vi "Gas_Release_Control.vi"(4 "Source Establishment Time (s)":dbl=20.0, 5 "Gas Line Name":T1, 6 "Strength (% by volume)":dbl format="%.3f", 7 "Carrier_2 Q (l/min)":dbl format="%.2f", 8 "Carrier_1 Q (l/min)":dbl format="%#.3f", 9 "Source Status":T3=enum."Using") -> (0 "error out":errorcluster, 1 "Flowrates (kg/min)":dbl[](array[numeric]) format="%.2f", 2 "Source Est Time (s)":dbl, 3 "Flowrates Achieved?":bool)   [LabVIEW 2022 SP3]
uses:
  ADAM Controls/Client_Source_Status.ctl
  ADAM Controls/Client_Source.ctl
  Anemometry/Anemometry Sub Vis/Controls/GMU Gas Line Name.ctl
  ADAM Controls/Channel_names.ctl
  ADAM Controls/Module_type_ADAM.ctl
  ADAM Controls/Channel_State.ctl
  ADAM Controls/Ch_description_ADAM.ctl
  ADAM Controls/Function_ADAM.ctl
  ADAM Controls/Calib_type_ADAM.ctl
  ADAM Controls/Address.ctl
  ADAM Controls/Update_scan_value.ctl
  Anemometry/Anemometry Sub Vis/Controls/In_Range.ctl
  Anemometry/Anemometry Sub Vis/Controls/Multi_run_mode.ctl
  Anemometry/Anemometry Sub Vis/Globals/Preference_global.vi
  Anemometry/Anemometry Sub Vis/Globals/Trav_pos_global.vi
  Anemometry/Anemometry Sub Vis/Globals/Gas_management_global.vi
panel:
  out "Q source":dbl
  out "Error String":string
  out "Current Case":T2=enum."Get Source Clients"
  out "Status of other Clients":string[](array[string])
  out "Source already correct?":bool
  out "No Other Clients are Using Source?":bool
  out "Source Clients":string[](array[string])
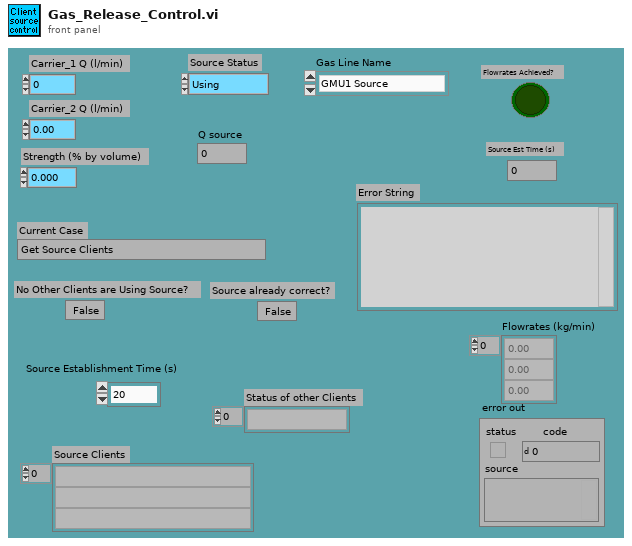
[diagram p1: front panel]
types:
  T1 = typedef "GMU Gas Line Name.ctl" = enum16{"GMU1 Source", "GMU2 Source", "GMU2 Calib", "CPP GRC-A", "CPP GRC-B"}
  T2 = typedef "Client_Source.ctl" = enum16{"Start", "Get Source Clients", "Has this client liberty to control the source?", "Declare not using, other client already waiting", "Is the Source already correct?", "Declare waiting, other client is still using", "Control Hi-Tec", "Were the Hi-tecs able to achieve the flowrates?", "Declare source status", "Wait for source to Establish"}
  T3 = typedef "Client_Source_Status.ctl" = enum16{"Not Using", "Using", "Must Have"}
  T4 = typedef "Channel_names.ctl" = enum16{"Active Only", "Active + Off", "All Channels", "Changeable Only"}
  T5 = typedef "Calib_type_ADAM.ctl" = string
  T6 = typedef "Ch_description_ADAM.ctl" = cluster{"Ch Name":string, "Type":T7, "Function":T8, "Ch State":T9, "Calibration type":T5, "A":dbl, "B":dbl, "C":dbl, "D":dbl, "Comments":string, "Address":T10, "String":string, "Duty":u16}
  T7 = typedef "Module_type_ADAM.ctl" = string
  T8 = typedef "Function_ADAM.ctl" = enum16{"Analogue Input", "Digital Input", "Event counter", "Event rate", "Analogue Output", "Digital Output", "Relay Output"}
  T9 = typedef "Channel_State.ctl" = enum16{"On", "Off", "Always On", "Always Off"}
  T10 = typedef "Address.ctl" = cluster{"Main":i32, "Ch.":i32, "Sub":i32, "Port Name":string}
  T11 = typedef "Update_scan_value.ctl" = cluster{"Channel Name":string, "New Value":dbl, "!Auto_Off":bool}
  T12 = typedef "In_Range.ctl" = enum16{"%", "±", "% & ±"}
  T13 = typedef "Multi_run_mode.ctl" = enum16{"Move Traverse Only", "Set Tunnel Speed Only", "Set Source Only", "Set Measurement Conditions", "Single Measurement", "Vertical Profile", "Lateral Profile", "Longitudinal Profile", "Multi-Axis Profile", "Explore Volume", "Auto Calibrate", "Meas Fast FID Bkgnd", "Check Beam Power", "Scanning Valve Measurement", "Run VI Named:", "Set ADAM Ch", "Wait (minutes)", "Send Message", "Synchronize With:", "Fall Back to this Row", "Turn Off Row Repeating", "Traverse 3D Volume", "Blank Row", "Jump to Fall Back Row"}
  T14 = typedef "Traverse_cluster.ctl" = cluster{"Start X":sgl, "Start Y":sgl, "Start Z":sgl, "End X":sgl, "End Y":sgl, "End Z":sgl, "nPoints":i32, "Spacing":T15, "Filename":path, "Tunnel Speed":dbl, "Averaging time (mins)":dbl, "Extra Commands":string, "Carrier_1 Q (l/min)":dbl, "Carrier_2 Q (l/min)":dbl, "Trace Gas Concentration (%)":dbl, "Specific Arguments":string, "Comments":string, "Row No":i32, "Row Type Selector":T13, "EstCompl":string, "Row Duration (mins)":dbl, "nValidPoints":i32, "Meas Setup File":string}
  T15 = typedef "Spacing.ctl" = enum16{"Linear", "Log", "Gauss", "Specified", "N/A"}
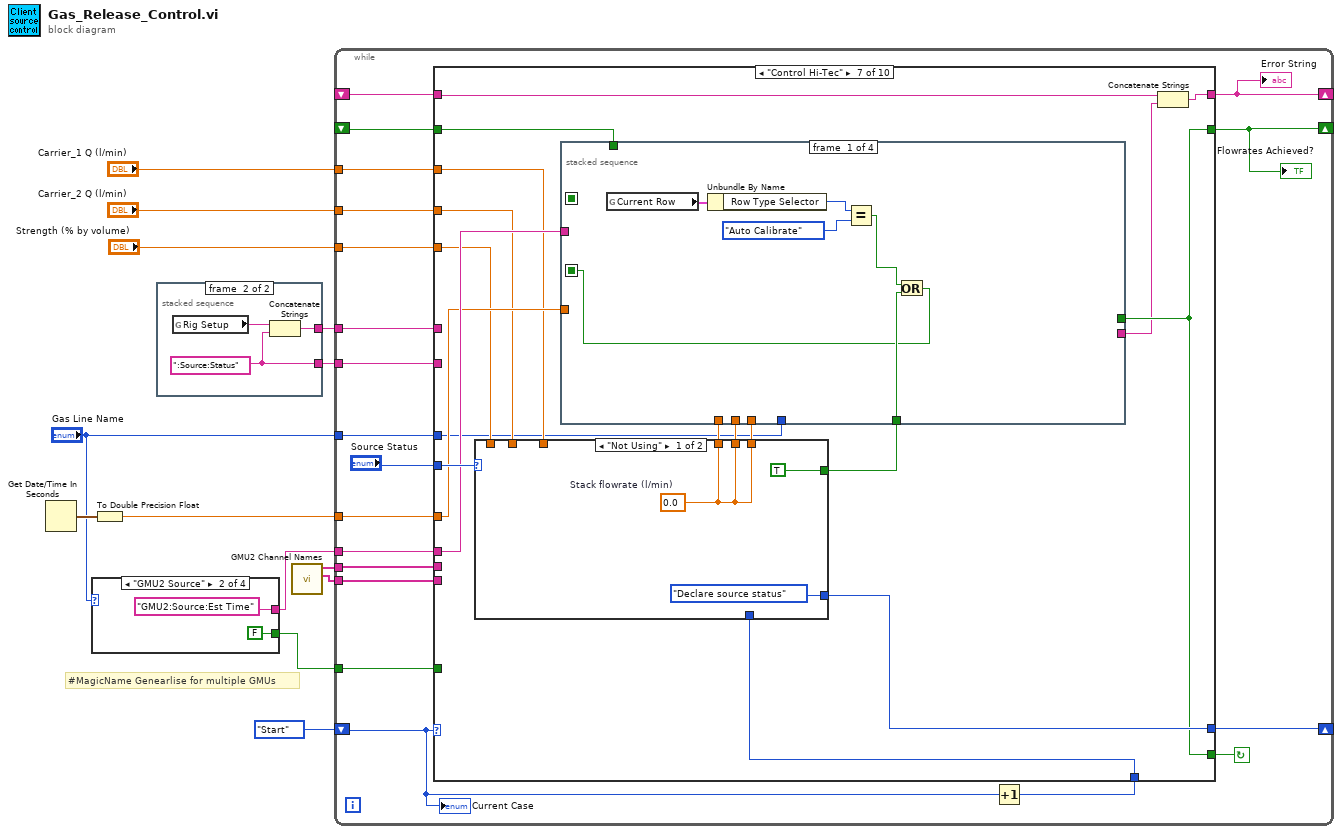
[diagram p0: block diagram]
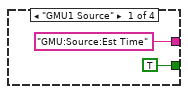
[diagram p2: hidden frame]
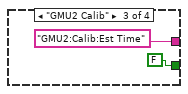
[diagram p3: hidden frame]
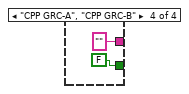
[diagram p4: hidden frame]
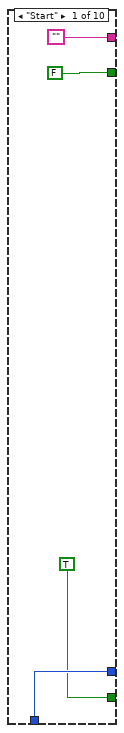
[diagram p5: hidden frame]
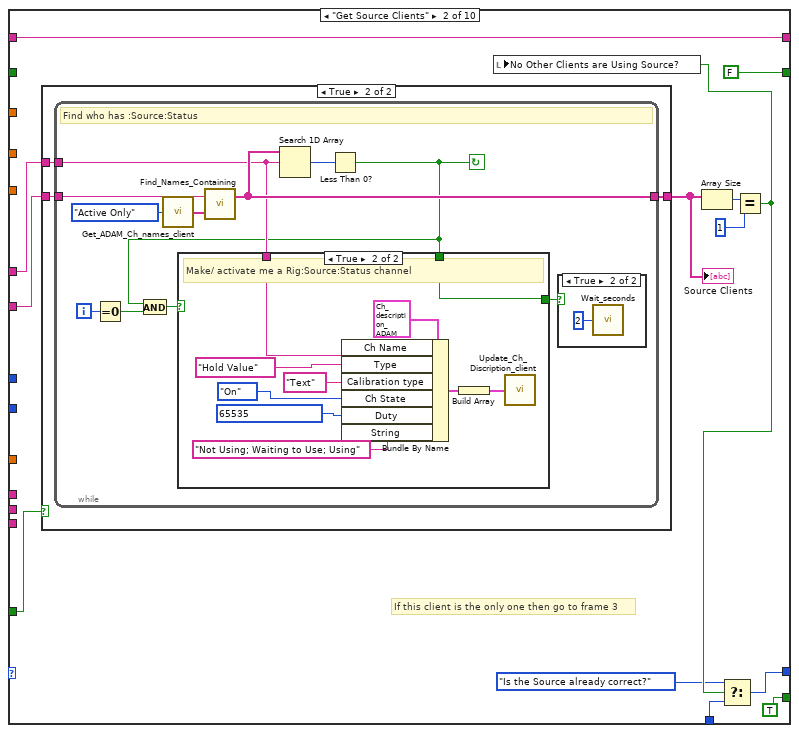
[diagram p6: hidden frame]
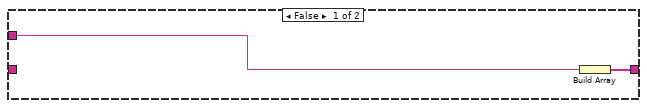
[diagram p7: hidden frame]
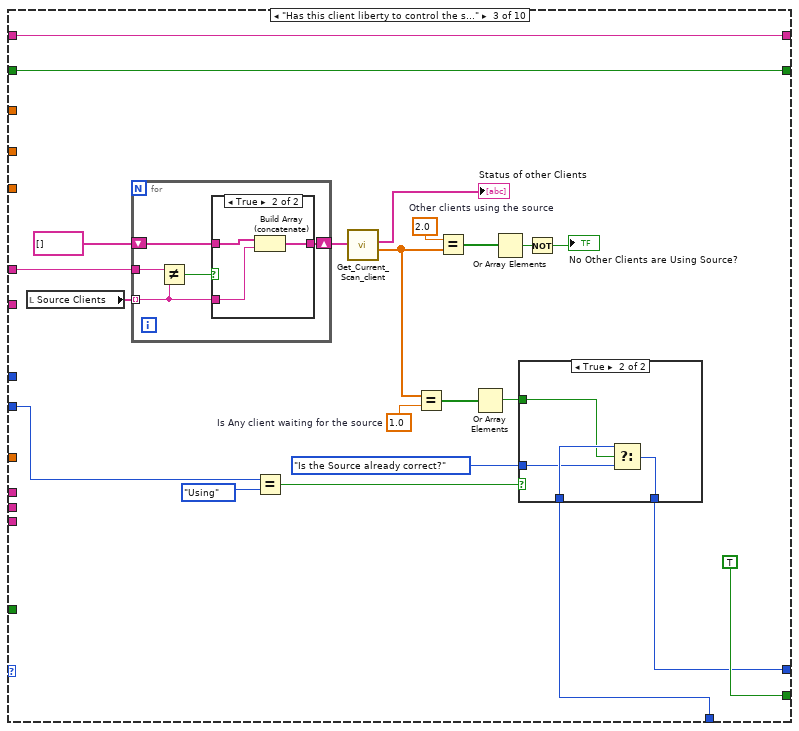
[diagram p10: hidden frame]
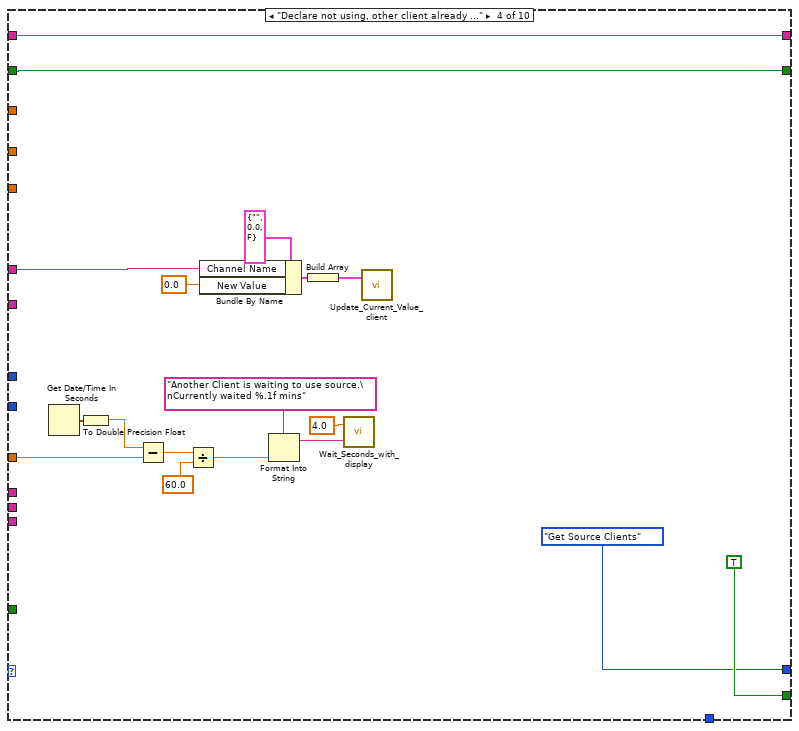
[diagram p13: hidden frame]
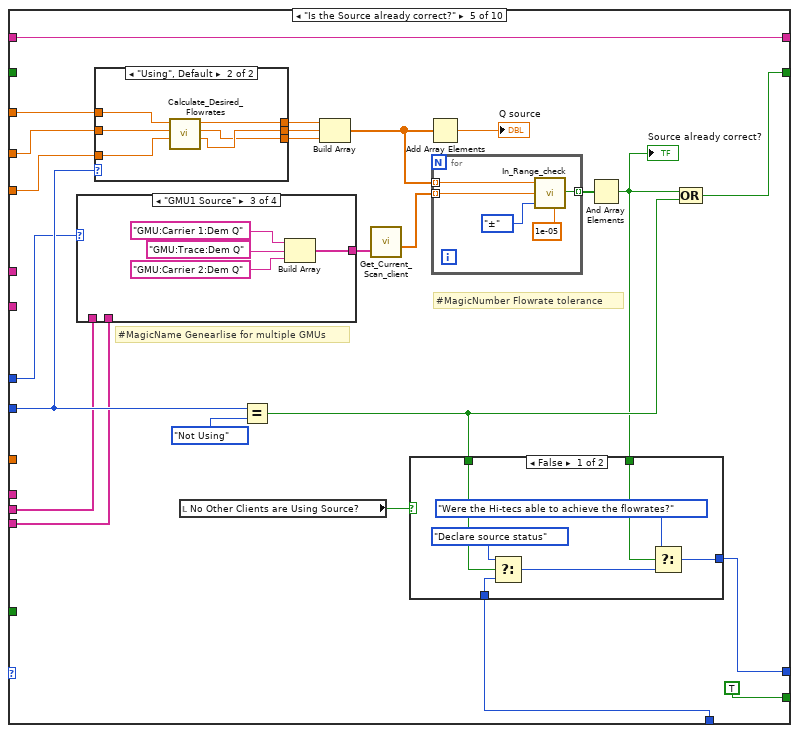
[diagram p14: hidden frame]
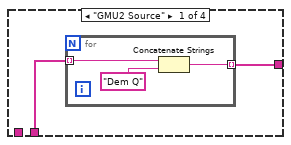
[diagram p15: hidden frame]
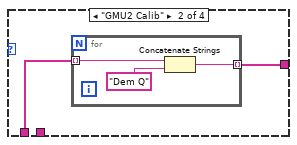
[diagram p16: hidden frame]
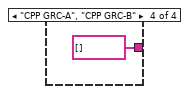
[diagram p17: hidden frame]
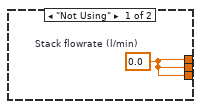
[diagram p18: hidden frame]
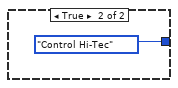
[diagram p19: hidden frame]
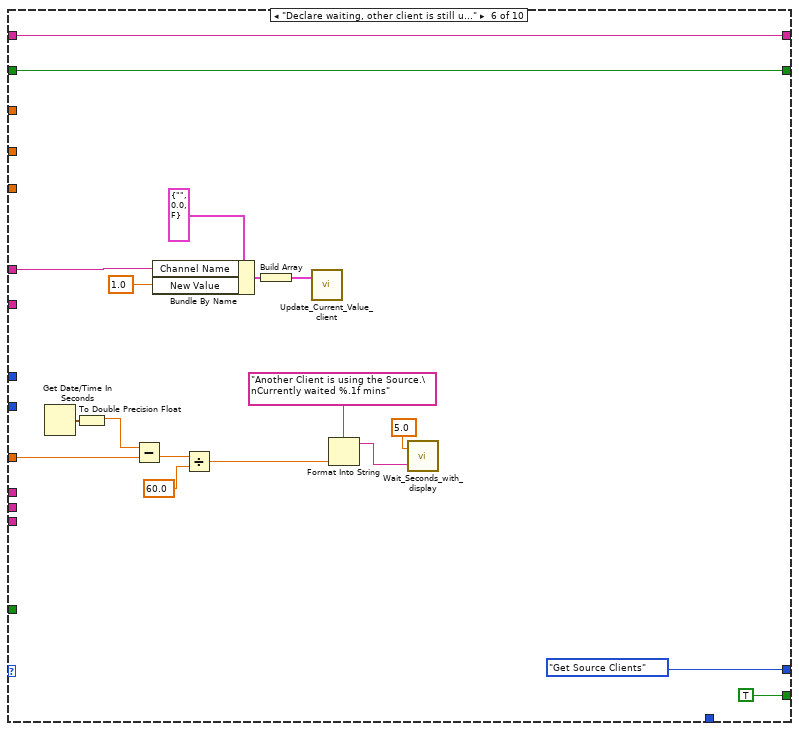
[diagram p20: hidden frame]
diagram:
  # "#MagicName Genearlise for multiple GMUs"
  n1 = Get Date/Time In Seconds() -> (seconds since 1Jan1904=w9:timestamp)
  n2 = case shown="\"GMU2 Source\"" "Gas Line Name" {
    tunnel: ["GMU:Source:Est Time" "GMU2:Source:Est Time" "GMU2:Calib:Est Time" ""] -> w8
    tunnel: [TRUE FALSE FALSE FALSE] -> w1
    frame "GMU1 Source" {
    }
    frame "GMU2 Source" {
    }
    frame "GMU2 Calib" {
    }
    frame "CPP GRC-A", "CPP GRC-B" {
    }
  }
  n3 = To Double Precision Float(number=w9) -> (double precision float=w11:dbl)
  n4 = stacked-sequence {
    tunnel: [_ w24] -> w13
    tunnel: [_ w23] -> w12
    frame #0 {
      n5 = call "Run_EnFlo_Hub.vi"() -> ()  [unwired: 1 in, 7 out]
    }
    frame #1 {
      w24 = ":Source:Status"
      n6 = global read "Preference_global.vi" "Rig Setup"() -> (w22:string)
      n7 = Concatenate Strings(w22, w24) -> (w23:string)
    }
  }
  n8 = call "GMU2 Channel Names.vi"() -> ("GMU2 Source Channels"=w3:string[], "GMU2 Calib Channels"=w2:string[])  [unwired: 10 in]
  n9 = while {
    tunnel: w11 -> [w40]
    tunnel: w12 -> [w43]
    shift-left: Client_Source."Start" -> [w38]
    shift-right: [w39] -> _
    tunnel: w13 -> [w44]
    shift-right: [w35] -> _
    shift-left: _ -> [w36]
    tunnel: w8 -> [w34]
    shift-right: [w32] -> _
    shift-left: _ -> [w33]
    tunnel: "Carrier_1 Q (l/min)" -> [w31]
    tunnel: "Carrier_2 Q (l/min)" -> [w30]
    tunnel: "Strength (% by volume)" -> [w29]
    tunnel: "Gas Line Name" -> [w28]
    tunnel: w3 -> [w27]
    tunnel: w2 -> [w26]
    tunnel: w1 -> [w25]
    stop <- w42 continue-if-true
    n10 = Increment(x=w38) -> (x+1=w41:T2)
    n11 = case shown="\"Control Hi-Tec\"" w38 {
      tunnel: w44 -> [_ w61 _ _ _ _ _ _ _ _]
      tunnel: [w48 w57 w104 Client_Source."Get Source Clients" w160 Client_Source."Get Source Clients" w235 w282 w403 w422] -> w39
      tunnel: w43 -> [_ w60 w111 w138 _ w215 _ _ w405 _]
      tunnel: [TRUE ("Establish Exp Conditions") TRUE TRUE TRUE TRUE TRUE w231 TRUE w397 FALSE] -> w42
      tunnel: w41 -> [w48 w56 w106 _ w165 _ w234 w280 w403 w422]
      tunnel: w40 -> [_ _ _ w136 _ w210 w232 _ _ _]
      tunnel: "Source Status" -> [_ _ w95 _ w163 _ w238 w290 w404 w418]
      tunnel: [FALSE FALSE w91 w128 w161 w205 w231 w289 w398 w421] -> w35
      tunnel: w36 -> [_ _ w91 w128 _ w205 w230 _ w398 w421]
      tunnel: w34 -> [_ _ _ _ _ _ w233 w287 _ _]
      tunnel: w33 -> [_ w50 w90 w126 w159 w203 w228 w286 w396 w420]
      tunnel: ["" w50 w90 w126 w159 w203 w229 w286 w395 w420] -> w32
      tunnel: w31 -> [_ _ _ _ w153 _ w226 _ _ _]
      tunnel: w30 -> [_ _ _ _ w152 _ w225 _ _ _]
      tunnel: w29 -> [_ _ _ _ w151 _ w224 _ _ w419]
      tunnel: w28 -> [_ _ _ _ w148 _ w222 w285 _ w417]
      tunnel: w27 -> [_ _ _ _ w145 _ _ w284 _ _]
      tunnel: w26 -> [_ _ _ _ w144 _ _ w283 _ _]
      tunnel: w25 -> [_ w49 _ _ _ _ _ w281 _ _]
      frame "Start" {
      }
      frame "Get Source Clients" {
        # "If this client is the only one then go to frame 3"
        n12 = case shown="True" w49 {
          tunnel: w61 -> [_ w66]
          tunnel: w60 -> [w63 w65]
          tunnel: [w62 w64] -> w54
          frame False {
            n13 = Build Array(w63) -> (w62:string[])
          }
          frame True {
            n14 = while {
              tunnel: [w70] -> w64
              tunnel: w65 -> [w69]
              tunnel: w66 -> [w77]
              i -> [w74]
              stop <- w67 continue-if-true
              # "Find who has :Source:Status"
              n15 = Equal To 0?(x=w74) -> (x = 0?=w73:bool)
              n16 = call "Get_ADAM_Ch_names_client.vi"("Channel names set"=Channel_names."Active Only") -> ("Ch names"=w75:string[])
              n17 = call "Find_Names_Containing.vi"("Ch names"=w75, "String to match"=w77) -> ("Matched Names"=w70:string[])  [unwired: 1 out]
              n18 = Search 1D Array(1D array=w70, element=w69) -> (index of element=w68:i32)  [unwired: 1 out]
              n19 = Less Than 0?(x=w68) -> (x < 0?=w67:bool)
              n20 = And(x=w67, y=w73) -> (x .and. y?=w72:bool)
              n21 = case shown="True" w72 {
                tunnel: w69 -> [_ w87]
                tunnel: [w79 w83] -> w71
                tunnel: w67 -> [w79 w83]
                frame False {
                }
                frame True {
                  # "Make/ activate me a Rig:Source:Status channel"
                  n22 = Bundle By Name(cluster=T6 {"Ch Name"="", "Type"="", "Function"=enum."Analogue Input", "Ch State"=enum."On", "Calibration type"="", "A"=0.0, "B"=0.0, "C"=0.0, "D"=0.0, "Comments"="", "Address"={"Main"=0, "Ch."=0, "Sub"=0, "Port Name"=""}, "String"="", "Duty"=65535} ("Ch Discription"), "Ch Name"=w87, "Type"=T7 "Hold Value", "Calibration type"=T5 "Text", "Ch State"=Channel_State."On", "Duty"=u16 65535 ("Bundle Element"), "String"="Not Using; Waiting to Use; Using") -> (w85:T6)
                  n23 = Build Array(w85) -> (w84:T6[])
                  n24 = call "Update_Ch_Discription_client.vi"("Channels to update In"=w84) -> ()  [unwired: 1 out]
                }
              }
              n25 = case shown="True" w71 {
                frame False {
                }
                frame True {
                  n26 = call "Wait_seconds.vi"("Seconds to wait"=u32 2) -> ()
                }
              }
            }
          }
        }
        "Source Clients" <- w54
        n27 = Array Size(array=w54) -> (size(s)=w59:i32)
        n28 = Equal?(x=w59, y=1) -> (x = y?=w53:bool)
        n29 = local write "No Other Clients are Using Source?"(w53) -> ()
        n30 = Select(t=Client_Source."Is the Source already correct?", s=w53, f=w56) -> (s? t:f=w57:T2)
      }
      frame "Has this client liberty to control the source?" {
        w103 = 2.0  # Other clients using the source
        w109 = 1.0  # Is Any client waiting for the source
        n31 = local read "Source Clients"() -> (w105:string[])
        n32 = for {
          tunnel: w105 -> [w117] mode=indexing
          tunnel: w111 -> [w121]
          shift-right: [w118] -> w101
          shift-left: string[] [] -> [w119]
          n33 = Not Equal?(x=w121, y=w117) -> (x != y?=w120:bool)
          n34 = case shown="True" w120 {
            tunnel: w119 -> [w122 w125]
            tunnel: [w122 w124] -> w118
            tunnel: w117 -> [_ w123]
            frame False {
            }
            frame True {
              n35 = Build Array (concatenate)(w125, w123) -> (w124:string[])
            }
          }
        }
        n36 = Equal?(x=w95, y=Client_Source_Status."Using" ("Source Status")) -> (x = y?=w94:bool)
        n37 = call "Get_Current_Scan_client.vi"("multipleChannels"=w101) -> ("String values"=→"Status of other Clients":string[], "Numerical Values"=w98:dbl[])  [unwired: 1 in, 2 out]
        n38 = Equal?(x=w98, y=w109) -> (x = y?=w108:bool[])
        n39 = Equal?(x=w103, y=w98) -> (x = y?=w102:bool[])
        n40 = Or Array Elements(Boolean array=w108) -> (logical OR=w99:bool)
        n41 = Or Array Elements(Boolean array=w102) -> (logical OR=w97:bool)
        n42 = case shown="True" w94 {
          tunnel: w106 -> [_ w116]
          tunnel: [w112 w115] -> w104
          tunnel: w99 -> [_ w114]
          tunnel: Client_Source."Is the Source already correct?" -> [w112 w113]
          frame False {
          }
          frame True {
            n43 = Select(t=w116, s=w114, f=w113) -> (s? t:f=w115:T2)
          }
        }
        n44 = Not(x=w97) -> (.not. x?=→"No Other Clients are Using Source?":bool)
      }
      frame "Declare not using, other client already waiting" {
        n45 = Get Date/Time In Seconds() -> (seconds since 1Jan1904=w127:timestamp)
        n46 = To Double Precision Float(number=w127) -> (double precision float=w137:dbl)
        n47 = Subtract(x=w137, y=w136) -> (x-y=w135:dbl)
        n48 = Divide(x=w135, y=60.0) -> (x/y=w129:dbl)
        n49 = Bundle By Name(cluster=T11 {"Channel Name"="", "New Value"=0.0, "!Auto_Off"=FALSE} ("Update Scan Value Cluster"), "Channel Name"=w138, "New Value"=0.0 ("Bundle Element")) -> (w141:T11)
        n50 = Format Into String(format string="Another Client is waiting to use source.\nCurrently waited %.1f mins" ("Format String"), w129) -> (resulting string=w132:string)  [unwired: 2 in, 1 out]
        n51 = Build Array(w141) -> (w140:T11[])
        n52 = call "Wait_Seconds_with_display.vi"("Message"=w132, "Seconds to wait"=4.0) -> ()  [unwired: 2 out]
        n53 = call "Update_Current_Value_client.vi"("Update array in"=w140) -> ()  [unwired: 1 in]
      }
      frame "Is the Source already correct?" {
        # "#MagicName Genearlise for multiple GMUs"
        # "#MagicNumber Flowrate tolerance"
        n54 = case shown="\"GMU1 Source\"" w148 {
          tunnel: [w168 w174 w178 string[] []] -> w147
          tunnel: w145 -> [w169 _ _ _]
          tunnel: w144 -> [_ w173 _ _]
          frame "GMU2 Source" {
            n55 = for {
              tunnel: w169 -> [w171] mode=indexing
              tunnel: [w170] -> w168 mode=indexing
              n56 = Concatenate Strings(w171, "Dem Q" ("string")) -> (w170:string)
            }
          }
          frame "GMU2 Calib" {
            n57 = for {
              tunnel: w173 -> [w176] mode=indexing
              tunnel: [w175] -> w174 mode=indexing
              n58 = Concatenate Strings(w176, "Dem Q" ("string")) -> (w175:string)
            }
          }
          frame "GMU1 Source" {
            n59 = Build Array("GMU:Carrier 1:Dem Q", "GMU:Trace:Dem Q", "GMU:Carrier 2:Dem Q") -> (w178:string[])
          }
          frame "CPP GRC-A", "CPP GRC-B" {
          }
        }
        n60 = case shown="\"Using\", Default" w163 {
          tunnel: [w188 w191] -> w158
          tunnel: [w188 w190] -> w157
          tunnel: [w188 w189] -> w156
          tunnel: w153 -> [_ w194]
          tunnel: w152 -> [_ w193]
          tunnel: w151 -> [_ w192]
          frame "Not Using" {
            w188 = 0.0  # Stack flowrate (l/min)
          }
          frame "Using", Default {
            n61 = call "Calculate_Desired_Flowrates.vi"("Strength (% by volume)"=w192, "Carrier_2 Q (l/min)"=w193, "Carrier_1 Q (l/min)"=w194) -> ("Trace Q l/min"=w190:dbl, "Carrier 2 l/min"=w189:dbl, "Carrier 1 l/min"=w191:dbl)  [unwired: 3 in, 2 out]
          }
        }
        n62 = local read "No Other Clients are Using Source?"() -> (w166:bool)
        n63 = Equal?(x=w163, y=Client_Source_Status."Not Using" ("Source Status")) -> (x = y?=w162:bool)
        n64 = Build Array(w158, w157, w156) -> (w150:dbl[])
        n65 = call "Get_Current_Scan_client.vi"("multipleChannels"=w147) -> ("Numerical Values"=w146:dbl[])  [unwired: 1 in, 3 out]
        n66 = Add Array Elements(numeric array=w150) -> (sum=→"Q source":dbl)
        n67 = for {
          tunnel: w146 -> [w185] mode=indexing
          tunnel: w150 -> [w184] mode=indexing
          tunnel: [w183] -> w155 mode=indexing
          n68 = call "In_Range_check.vi"("±"=1e-05, "Mode"=In_Range."±", "Value"=w185, "Setpoint"=w184) -> ("In Range"=w183:bool)  [unwired: 1 in, 2 out]
        }
        n69 = And Array Elements(Boolean array=w155) -> (logical AND=w154:bool)
        "Source already correct?" <- w154
        n70 = case shown="False" w166 {
          tunnel: w165 -> [w201 _]
          tunnel: w162 -> [w200 _]
          tunnel: w154 -> [w198 _]
          tunnel: [w196 Client_Source."Control Hi-Tec"] -> w160
          frame False {
            n71 = Select(t=Client_Source."Declare source status", s=w200, f=w201) -> (s? t:f=w197:T2)
            n72 = Select(t=Client_Source."Were the Hi-tecs able to achieve the flowrates?", s=w198, f=w197) -> (s? t:f=w196:T2)
          }
          frame True {
          }
        }
        n73 = Compound Arithmetic op=OR(w154, w162) -> (w161:bool)
      }
      frame "Declare waiting, other client is still using" {
        n74 = Get Date/Time In Seconds() -> (seconds since 1Jan1904=w204:timestamp)
        n75 = To Double Precision Float(number=w204) -> (double precision float=w213:dbl)
        n76 = Subtract(x=w213, y=w210) -> (x-y=w212:dbl)
        n77 = Bundle By Name(cluster=T11 {"Channel Name"="", "New Value"=0.0, "!Auto_Off"=FALSE} ("Update Scan Value Cluster"), "Channel Name"=w215, "New Value"=1.0 ("Bundle Element")) -> (w218:T11)
        n78 = Divide(x=w212, y=60.0) -> (x/y=w206:dbl)
        n79 = Build Array(w218) -> (w217:T11[])
        n80 = call "Update_Current_Value_client.vi"("Update array in"=w217) -> ()  [unwired: 1 in]
        n81 = Format Into String(format string="Another Client is using the Source.\nCurrently waited %.1f mins" ("Format String"), w206) -> (resulting string=w209:string)  [unwired: 2 in, 1 out]
        n82 = call "Wait_Seconds_with_display.vi"("Message"=w209, "Seconds to wait"=5.0) -> ()  [unwired: 2 out]
      }
      frame "Control Hi-Tec" {
        n83 = case shown="\"Not Using\"" w238 {
          tunnel: [w272 w278] -> w237
          tunnel: w226 -> [_ w278]
          tunnel: [w272 w277] -> w236
          tunnel: w225 -> [_ w277]
          tunnel: [Client_Source."Declare source status" w276] -> w235
          tunnel: w234 -> [_ w276]
          tunnel: w224 -> [_ w275]
          tunnel: [w272 w275] -> w223
          tunnel: [TRUE FALSE] -> w221
          frame "Not Using" {
            w272 = 0.0  # Stack flowrate (l/min)
          }
          frame "Using", Default {
          }
        }
        n84 = stacked-sequence {
          seq-local: [_ _ _ w264] -> [_ _ _ _]
          seq-local: [w239 _ _ _] -> [_ _ w252 _]
          tunnel: w237 -> [_ _ _ w268]
          tunnel: w236 -> [_ _ _ w267]
          tunnel: w233 -> [_ w245 _ _]
          tunnel: w232 -> [_ _ _ _]
          tunnel: [_ _ _ w264] -> w231
          tunnel: w230 -> [_ w246 _ _]
          tunnel: [_ _ _ w263] -> w227
          tunnel: w223 -> [_ _ _ w262]
          tunnel: w222 -> [_ _ _ w261]
          tunnel: w221 -> [w240 _ _ _]
          frame #0 {
            n85 = global read "Trav_pos_global.vi" "Current Row"() -> (w244:T14)
            n86 = Unbundle By Name(w244) -> ("Row Type Selector"=w243:T13)
            n87 = Equal?(x=w243, y=Multi_run_mode."Auto Calibrate" ("Row Type Selector")) -> (x = y?=w241:bool)
            n88 = Or(x=w241, y=w240) -> (x .or. y?=w239:bool)
          }
          frame #1 {
            n89 = case shown="False" w246 {
              tunnel: w245 -> [w248 _]
              frame False {
                n90 = Bundle By Name(cluster=T11 {"Channel Name"="", "New Value"=0.0, "!Auto_Off"=FALSE} ("Update Scan Value Cluster"), "Channel Name"=w248, "New Value"=0.0) -> (w250:T11)
                n91 = Build Array(w250) -> (w249:T11[])
                n92 = call "Update_Current_Value_client.vi"("Update array in"=w249) -> ()  [unwired: 1 in]
              }
              frame True {
              }
            }
          }
          frame #2 {
            n93 = case shown="True" w252 {
              frame False {
                n94 = call "Is Puff_using_Arduino Plugin used"() -> ("Puff_using_Arduino.vi"=w253:bool)  [unwired: 1 in]
                n95 = case shown="True" w253 {
                  frame True {
                    w256 = u32 1  # Time to hold source OFF (microseconds)
                    w255 = u32 0  # Time to hold source ON (microseconds)
                    n96 = call "Arduino_Timed_Release.vi"("Time to hold source ON (microseconds)"=w255, "Time to hold source OFF (microseconds)"=w256, "Number of cycles"=u16 1) -> ()  [unwired: 2 out]
                  }
                  frame False {
                    n97 = global read "Gas_management_global.vi" "Source Live"() -> (w257:bool)
                    n98 = case shown="False" w257 {
                      frame False {
                        w260 = u32 0  # Time to hold source OFF (microseconds)
                        w259 = u32 1  # Time to hold source ON (microseconds)
                        n99 = call "Arduino_Timed_Release.vi"("Time to hold source ON (microseconds)"=w259, "Time to hold source OFF (microseconds)"=w260, "Number of cycles"=u16 1) -> ()  [unwired: 2 out]
                      }
                      frame True {
                      }
                    }
                  }
                }
              }
              frame True {
              }
            }
          }
          frame #3 {
            n100 = call "Set_Hi-Tec_client.vi"("Gas Line Name"=w261, "Strength (% by volume)"=w262, "Carrier_2 Q (l/min)"=w267, "Carrier_1 Q (l/min)"=w268, "Mode"=enum16{"Control Hi-Tec", "Check Hi-Tec Demands"}."Control Hi-Tec") -> ("error out"=w266:errorcluster, "Flowrates (kg/min)"=→"Flowrates (kg/min)":dbl[])  [unwired: 1 in, 2 out]
            "error out" <- w266
            n101 = Unbundle By Name(w266) -> ("status"=w265:bool, "source"=w263:string)
            n102 = Not(x=w265) -> (.not. x?=w264:bool)
          }
        }
        n103 = Concatenate Strings(w228, w227) -> (w229:string)
      }
      frame "Were the Hi-tecs able to achieve the flowrates?" {
        n104 = Get Date/Time In Seconds() -> (seconds since 1Jan1904=w288:timestamp)
        n105 = To Double Precision Float(number=w288) -> (double precision float=w291:dbl)
        n106 = while {
          tunnel: w290 -> [w301]
          tunnel: w291 -> [w305]
          tunnel: [w300] -> w289
          tunnel: w287 -> [w298]
          tunnel: w285 -> [w296]
          tunnel: w284 -> [w295]
          tunnel: w283 -> [w294]
          stop <- w302 continue-if-true
          n107 = case shown="\"GMU1 Source\"" w296 {
            tunnel: w301 -> [w319 w332 w364 _]
            tunnel: [w317 w331 w363 FALSE] -> w300
            tunnel: w298 -> [w316 w329 w361 _]
            tunnel: w295 -> [_ _ w362 _]
            tunnel: w294 -> [_ w330 _ _]
            tunnel: [w307 w328 w360 0.0] -> w293
            frame "GMU1 Source" {
              w308 = 20.0  # %
              w323 = 1.0  # %
              n108 = case shown="\"Using\", Default" w319 {
                tunnel: [w326 w327] -> w309
                frame "Not Using" {
                  w326 = 0.0  # Stack flowrate (l/min)
                }
                frame "Using", Default {
                  n109 = local read "Q source"() -> (w327:dbl)
                }
              }
              n110 = Build Array("GMU:Source:Dem Q", w316, "GMU:Source:Meas Q") -> (w325:string[])
              n111 = call "Get_Current_Scan_client.vi"("multipleChannels"=w325) -> ("Numerical Values"=w321:dbl[])  [unwired: 1 in, 3 out]
              n112 = Index Array(array=w321) -> (element #1=w312:dbl, element #2=w307:dbl, element #3=w313:dbl)  [unwired: 3 in]
              n113 = call "In_Range_check.vi"("%"=w308, "Mode"=In_Range."%", "Value"=w313, "Setpoint"=w309) -> ("In Range"=w310:bool)  [unwired: 1 in, 2 out]
              n114 = Greater Than 0?(x=w307) -> (x > 0?=w311:bool)
              n115 = call "In_Range_check.vi"("±"=0.1, "%"=w323, "Mode"=In_Range."% & ±", "Value"=w312, "Setpoint"=w309) -> ("In Range"=w320:bool)  [unwired: 2 out]
              n116 = Compound Arithmetic op=AND(w320, w310, w311) -> (w317:bool)
            }
            frame "GMU2 Calib" {
              n117 = case shown="\"Not Using\", Default" w332 {
                tunnel: [TRUE w340] -> w331
                tunnel: w330 -> [_ w339]
                tunnel: w329 -> [_ w336]
                tunnel: [0.0 w335] -> w328
                frame "Not Using", Default {
                }
                frame "Using" {
                  w346 = 20.0  # %
                  w351 = 20.0  # %
                  n118 = for {
                    tunnel: w339 -> [w357] mode=indexing
                    tunnel: [w354] -> w338 mode=concatenating
                    n119 = Concatenate Strings(w357, "Meas Volts" ("string")) -> (w356:string)
                    n120 = Concatenate Strings(w357, "Dem Volts" ("string")) -> (w355:string)
                    n121 = Build Array(w355, w356) -> (w354:string[])
                  }
                  n122 = Build Array (concatenate)(w338, w336) -> (w337:string[])
                  n123 = call "Get_Current_Scan_client.vi"("multipleChannels"=w337) -> ("Numerical Values"=w353:dbl[])  [unwired: 1 in, 3 out]
                  n124 = Index Array(array=w353) -> (element #1=w350:dbl, element #2=w349:dbl, element #3=w344:dbl, element #4=w343:dbl, element #5=w335:dbl)  [unwired: 5 in]
                  n125 = call "In_Range_check.vi"("±"=0.05, "%"=w351, "Mode"=In_Range."% & ±", "Value"=w349, "Setpoint"=w350) -> ("In Range"=w341:bool)  [unwired: 2 out]
                  n126 = call "In_Range_check.vi"("±"=0.05, "%"=w346, "Mode"=In_Range."% & ±", "Value"=w343, "Setpoint"=w344) -> ("In Range"=w342:bool)  [unwired: 2 out]
                  n127 = And(x=w341, y=w342) -> (x .and. y?=w340:bool)
                }
              }
            }
            frame "GMU2 Source" {
              n128 = case shown="\"Using\"" w364 {
                tunnel: [TRUE w372] -> w363
                tunnel: w362 -> [_ w371]
                tunnel: w361 -> [_ w370]
                tunnel: [0.0 w367] -> w360
                frame "Not Using", Default {
                }
                frame "Using" {
                  w378 = 20.0  # %
                  w383 = 20.0  # %
                  n129 = for {
                    tunnel: w371 -> [w389] mode=indexing
                    tunnel: [w386] -> w369 mode=concatenating
                    n130 = Concatenate Strings(w389, "Meas Volts" ("string")) -> (w388:string)
                    n131 = Concatenate Strings(w389, "Dem Volts" ("string")) -> (w387:string)
                    n132 = Build Array(w387, w388) -> (w386:string[])
                  }
                  n133 = Build Array (concatenate)(w369, w370) -> (w368:string[])
                  n134 = call "Get_Current_Scan_client.vi"("multipleChannels"=w368) -> ("Numerical Values"=w385:dbl[])  [unwired: 1 in, 3 out]
                  n135 = Index Array(array=w385) -> (element #1=w382:dbl, element #2=w381:dbl, element #3=w376:dbl, element #4=w375:dbl, element #5=w367:dbl)  [unwired: 5 in]
                  n136 = call "In_Range_check.vi"("±"=0.05, "%"=w383, "Mode"=In_Range."% & ±", "Value"=w381, "Setpoint"=w382) -> ("In Range"=w373:bool)  [unwired: 2 out]
                  n137 = call "In_Range_check.vi"("±"=0.05, "%"=w378, "Mode"=In_Range."% & ±", "Value"=w375, "Setpoint"=w376) -> ("In Range"=w374:bool)  [unwired: 2 out]
                  n138 = And(x=w373, y=w374) -> (x .and. y?=w372:bool)
                }
              }
            }
            frame "CPP GRC-A", "CPP GRC-B" {
            }
          }
          "Source Est Time (s)" <- w293
          n139 = Get Date/Time In Seconds() -> (seconds since 1Jan1904=w299:timestamp)
          n140 = To Double Precision Float(number=w299) -> (double precision float=w306:dbl)
          n141 = Subtract(x=w306, y=w305) -> (x-y=w297:dbl)
          n142 = Less?(x=w297, y=50.0) -> (x < y?=w303:bool)
          n143 = Compound Arithmetic op=AND(invert w300, w303) -> (w302:bool)
          n144 = case shown="True" w302 {
            frame False {
            }
            frame True {
              n145 = Wait (ms)(milliseconds to wait=u32 1000) -> ()  [unwired: 1 out]
            }
          }
        }
        n146 = Increment(x=w280) -> (x+1=w279:T2)
        n147 = Select(t=w280, s=w281, f=w279) -> (s? t:f=w282:T2)
      }
      frame "Declare source status" {
        n148 = case shown="True" w398 {
          tunnel: w404 -> [_ w414]
          tunnel: [0.0 w413] -> w399
          tunnel: [FALSE TRUE] -> w397
          tunnel: w396 -> [w407 w412]
          tunnel: [w406 w412] -> w395
          frame False {
            n149 = Concatenate Strings(w407, "Requested Flowrate has not been acheived.\n" ("Error String")) -> (w406:string)
          }
          frame True {
            n150 = case shown="\"Using\", \"Must Have\"" w414 {
              tunnel: [0.0 2.0] -> w413
              frame "Not Using" {
              }
              frame "Using", "Must Have" {
              }
            }
          }
        }
        n151 = Bundle By Name(cluster=T11 {"Channel Name"="", "New Value"=0.0, "!Auto_Off"=FALSE} ("Update Scan Value Cluster"), "Channel Name"=w405, "New Value"=w399) -> (w401:T11)
        n152 = Build Array(w401) -> (w400:T11[])
        n153 = call "Update_Current_Value_client.vi"("Update array in"=w400) -> ()  [unwired: 1 in]
      }
      frame "Wait for source to Establish" {
        n154 = case shown="\"Not Using\"" w418 {
          tunnel: w419 -> [_ w433]
          tunnel: w417 -> [_ w429]
          frame "Not Using" {
            n155 = global read "Gas_management_global.vi" "Source Live"() -> (w424:bool)
            n156 = case shown="True" w424 {
              frame False {
              }
              frame True {
                w427 = u32 1  # Time to hold source OFF (microseconds)
                w426 = u32 0  # Time to hold source ON (microseconds)
                n157 = call "Arduino_Timed_Release.vi"("Time to hold source ON (microseconds)"=w426, "Time to hold source OFF (microseconds)"=w427, "Number of cycles"=u16 1) -> ()  [unwired: 2 out]
              }
            }
          }
          frame "Using", "Must Have" {
            w439 = 4.0  # Number of Purges
            # "#MagicNumber Volume of stack tubing"
            n158 = local read "Q source"() -> (w430:dbl)
            n159 = case shown="\"GMU2 Calib\"" w429 {
              tunnel: [w450 w451 w452 w453 w454] -> w441
              frame "GMU1 Source" {
                w450 = 0.9  # Volume to flush (Litres)
              }
              frame "GMU2 Source" {
                w451 = 0.2  # Volume to flush (Litres)
              }
              frame "GMU2 Calib" {
                w452 = 0.2  # Volume to flush (Litres)
              }
              frame "CPP GRC-A" {
                w453 = 0.24  # Volume to flush (Litres)
              }
              frame "CPP GRC-B" {
                w454 = 0.24  # Volume to flush (Litres)
              }
            }
            n160 = local read "Source Est Time (s)"() -> (w445:dbl)
            n161 = Equal To 0?(x=w430) -> (x = 0?=w435:bool)
            n162 = Not A Number/Path/Refnum?(number/path/refnum=w445) -> (NaN/Path/Refnum?=w447:bool)
            n163 = Equal?(x=w433, y=100.0) -> (x = y?=w432:bool)
            n164 = Or(x=w435, y=w432) -> (x .or. y?=w431:bool)
            n165 = Divide(x=w441, y=w430) -> (x/y=w440:dbl)
            n166 = Multiply(x=w439, y=w440) -> (x*y=w438:dbl)
            n167 = Multiply(x=w438, y=60.0) -> (x*y=w436:dbl)
            n168 = Select(t=0.0, s=w431, f=w436) -> (s? t:f=w442:dbl)
            n169 = Add(x=w442, y="Source Establishment Time (s)") -> (x+y=w444:dbl)
            n170 = Subtract(x=w444, y=w445) -> (x-y=w446:dbl)
            n171 = Greater Than 0?(x=w446) -> (x > 0?=w449:bool)
            n172 = Or(x=w449, y=w447) -> (x .or. y?=w448:bool)
            n173 = case shown="True" w448 {
              tunnel: w447 -> [_ w459]
              tunnel: w444 -> [_ w458]
              tunnel: w446 -> [_ w457]
              frame False {
              }
              frame True {
                n174 = Select(t=w458, s=w459, f=w457) -> (s? t:f=w456:dbl)
                n175 = call "Wait_Seconds_with_display.vi"("Message"="Establishing Source", "Seconds to wait"=w456) -> ()  [unwired: 1 in, 1 out]
              }
            }
          }
        }
      }
    }
    "Flowrates Achieved?" <- w35
    "Error String" <- w32
    "Current Case" <- w38
  }
